vi "Phasor Explorer Update Parameters.vi"(8 "error in (no error)":errorcluster, 11 "VI in":refnum<vi>) -> (0 "error out":errorcluster, 1 "Detector Parameters":T12={"Frames/Image"=0, "Gates/Frame"=1, "Bits/Frame"=1, "Multiplicity"=0, "Incident Signal"=0.0, "Poisson Signal"=FALSE} {"Frames/Image" min=1; "Multiplicity" min=0; "Bits/Frame" min=1; "Gates/Frame" min=1}, 2 "Display Parameters":T10={"# Points"=1, "Ramp Type"=enum."Linear", "Type of Series"=enum."1-Exp Decays", "Min tau"=0.0, "Max tau"=0.0, "Include 0"=FALSE, "Include Infinity"=FALSE} {"Min tau" min=0.0; "Max tau" min=0.0; "# Points" min=1 step=1}, 3 "Decay & IRF Parameters":T8 {"Lifetime" min=0.0; "IRF Period" min=0.0}, 4 "tau*":dbl[unit], 5 "Gate Parameters":T5={"First Gate Start"=0.0, "Use Gate Center"=FALSE, "Gate Width"=0.0, "Gate Step"=0.0, "# Gates"=1.0, "Gate Type"=enum."Square", "Edge Width"=0.0, "Top Slope"=0.0, "Reversed Sawtooth?"=FALSE, "Analytical Computation"=FALSE, "Integration"=enum."Item 0", "Tolerance"=1.0, "# Steps"=1.0, "Type of User-defined Function"=enum."Gate", "Use Gate Step"=FALSE} {"# Steps" min=0.0; "Tolerance" min=0.0; "Top Slope" min=0.0; "Edge Width" min=0.0; "Gate Step" min=0.0; "# Gates" min=1.0 step=1.0; "Gate Width" min=0.0}, 6 "f0":dbl[unit], 7 "Phasor Parameters":T2={"Harmonic Frequency"=0.0, "Use f* = 1/D Frequency"=FALSE, "Calibrated Phasor"=FALSE, "Calibration Lifetime"=1e-09, "Phasor Calculation"=enum."Direct Sum", "SEPL Type"=enum."UC", "# Gates"=1.0, "Square Gate Width"=1e-09, "Show Ticks"=FALSE} {"Square Gate Width" min=0.0; "# Gates" min=0.0; "Calibration Lifetime" min=0.0; "Harmonic Frequency" min=0.0})   [LabVIEW 2019]
uses:
  Phasor Explorer Gate Parameter to Adjust.ctl
  Phasor Explorer Phasor Parameters.ctl
  Phasor Calculation Type.ctl
  SEPL Type.ctl
  Phasor Explorer Gate Parameters.ctl
  Gate Type.ctl
  Type of User-defined Function.ctl
  Phasor Explorer Decay Parameters.ctl
  IRF Model.ctl
  Phasor Explorer Display Parameters.ctl
  Type of Series.ctl
  Phasor Explorer Detector Parameters.ctl
panel:
  in  "Tab Control":T1(tab)
  in  "Edit User-defined Gate":bool
  in  "Gate Parameter to Adjust":T13 caption="Parameter to adjust"
  in  "Match Laser Period":bool
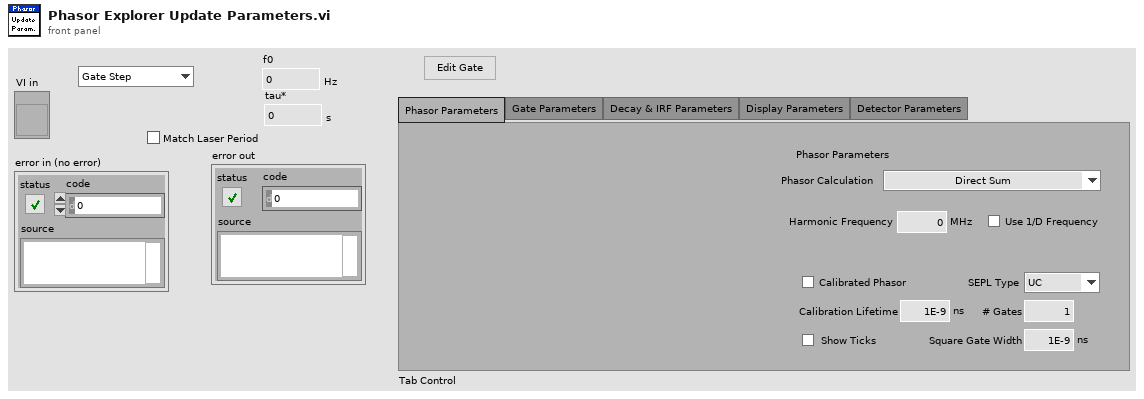
[diagram p1: front panel]
types:
  T1 = enum32{"Phasor Parameters", "Gate Parameters", "Decay & IRF Parameters", "Display Parameters", "Detector Parameters"}
  T2 = typedef "Phasor Explorer Phasor Parameters.ctl" = cluster{"Harmonic Frequency":dbl[unit], "Use f* = 1/D Frequency":bool, "Calibrated Phasor":bool, "Calibration Lifetime":dbl[unit], "Phasor Calculation":T3, "SEPL Type":T4, "# Gates":dbl, "Square Gate Width":dbl[unit], "Show Ticks":bool}
  T3 = typedef "Phasor Calculation Type.ctl" = enum16{"Direct Sum", "Analytical Formula"}
  T4 = typedef "SEPL Type.ctl" = enum16{"UC", "L_N", "L_N[W]", "L_X"}
  T5 = typedef "Phasor Explorer Gate Parameters.ctl" = cluster{"First Gate Start":dbl[unit], "Use Gate Center":bool, "Gate Width":dbl[unit], "Gate Step":dbl[unit], "# Gates":dbl, "Gate Type":T6, "Edge Width":dbl[unit], "Top Slope":dbl[unit], "Reversed Sawtooth?":bool, "Analytical Computation":bool, "Integration":enum32{"Item 0", "Item 1"}, "Tolerance":dbl, "# Steps":dbl, "Type of User-defined Function":T7, "Use Gate Step":bool}
  T6 = typedef "Gate Type.ctl" = enum16{"Square", "Finite Edge Square", "Finite Edge, Tilted Top Square", "Triangle", "Sawtooth", "User-defined"}
  T7 = typedef "Type of User-defined Function.ctl" = enum16{"Gate", "IRF"}
  T8 = typedef "Phasor Explorer Decay Parameters.ctl" = cluster{"Lifetime":dbl[unit], "IRF Offset":dbl[unit], "IRF Period":dbl[unit], "Normalized Decays":bool, "IRF Model":T9, "IRF Parameter 1":dbl[unit]}
  T9 = typedef "IRF Model.ctl" = enum16{"Dirac", "Exponential"}
  T10 = typedef "Phasor Explorer Display Parameters.ctl" = cluster{"# Points":i32, "Ramp Type":enum16{"Linear", "Logarithmic"}, "Type of Series":T11, "Min tau":dbl[unit], "Max tau":dbl[unit], "Include 0":bool, "Include Infinity":bool}
  T11 = typedef "Type of Series.ctl" = enum16{"1-Exp Decays", "Linear Combination of 1-Exp"}
  T12 = typedef "Phasor Explorer Detector Parameters.ctl" = cluster{"Frames/Image":i32, "Gates/Frame":i32, "Bits/Frame":i32, "Multiplicity":i32, "Incident Signal":dbl, "Poisson Signal":bool}
  T13 = typedef "Phasor Explorer Gate Parameter to Adjust.ctl" = enum16{"Gate Step", "# Gates"}
  T14 = typedef "SEPXP Gate Parameter to Adjust.ctl" = enum16{"Gate Step", "# Gates"}
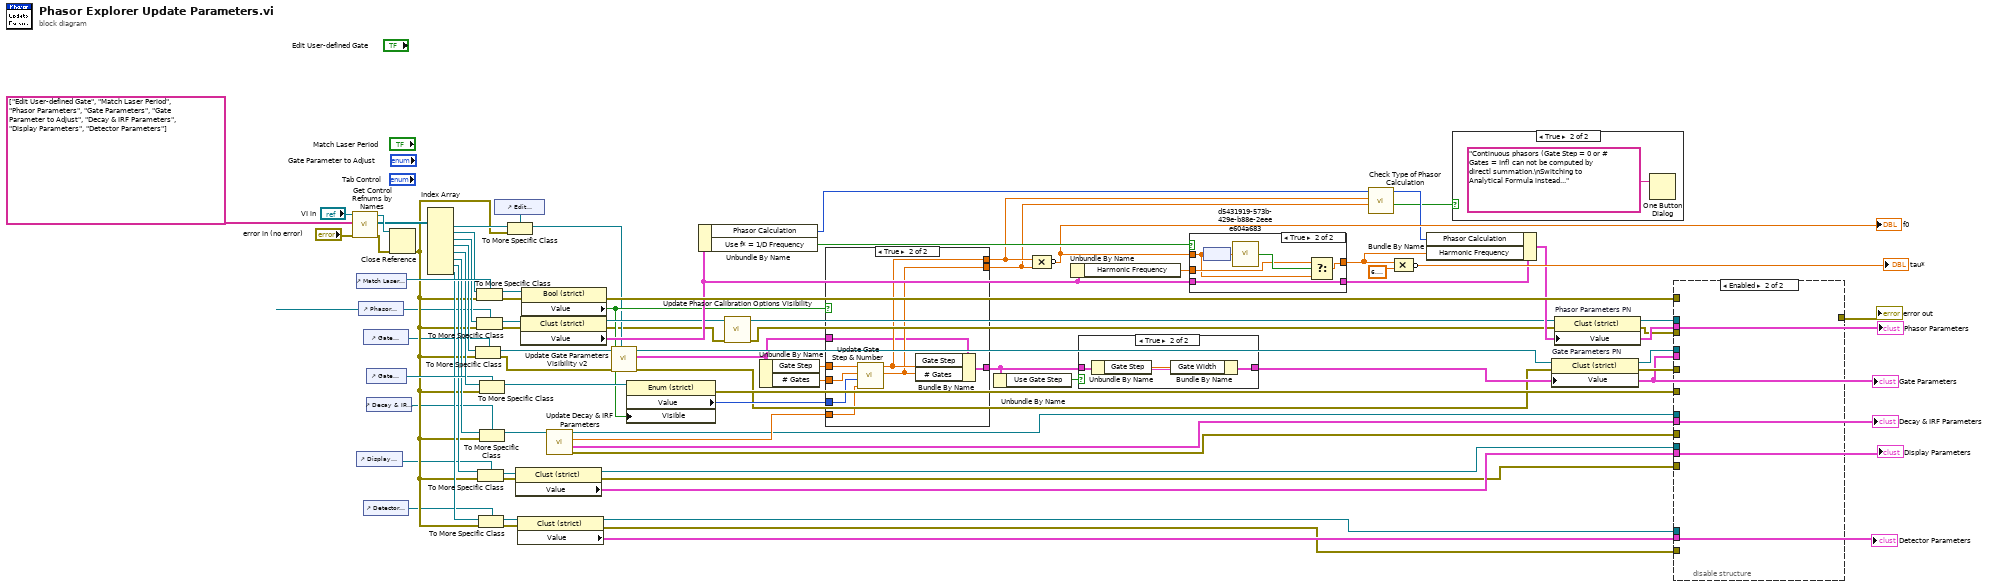
[diagram p0: block diagram]
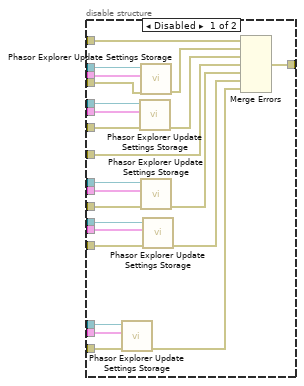
[diagram p2: hidden frame]
diagram:
  n1 = call "Get Control Refnums by Names.vi"("error in"="error in (no error)", "Control Labels"=string[] ["Edit User-defined Gate", "Match Laser Period", "Phasor Parameters", "Gate Parameters", "Gate Parameter to Adjust", "Decay & IRF Parameters", "Display Parameters", "Detector Parameters"], "VI  Ref"="VI in") -> ("error out"=w26:errorcluster, "Ctl Refnums"=w77:refnum<vi>[], "VI  Ref (out)"=w78:refnum<vi>)  [unwired: 5 in, 1 out]
  n2 = control-ref of="Match Laser Period"() -> (w72:refnum<vi>)
  n3 = control-ref of="Display Parameters"() -> (w6:refnum<vi>)
  n4 = control-ref of="Phasor Parameters"() -> (w9:refnum<vi>)
  n5 = control-ref of="Gate Parameters"() -> (w8:refnum<vi>)
  n6 = control-ref of="Detector Parameters"() -> (w5:refnum<vi>)
  n7 = control-ref of="Gate Parameter to Adjust"() -> (w66:refnum<vi>)
  n8 = control-ref of="Decay & IRF Parameters"() -> (w7:refnum<vi>)
  n9 = Close Reference(reference=w78, error in (no error)=w26) -> (error out=w21:errorcluster)
  n10 = Index Array(array=w77) -> (element #1=w25:refnum<vi>, element #2=w57:refnum<vi>, element #3=w56:refnum<vi>, element #4=w55:refnum<vi>, element #5=w68:refnum<vi>, element #6=w54:refnum<vi>, element #7=w41:refnum<vi>, element #8=w22:refnum<vi>)  [unwired: 8 in]
  n11 = To More Specific Class(target class=w8, reference=w55, error in=w21) -> (specific class reference=w61:refnum<vi>, error out=w60:errorcluster)
  n12 = To More Specific Class(target class=w72, reference=w57, error in=w21) -> (specific class reference=w71:refnum<vi>, error out=w70:errorcluster)
  n13 = To More Specific Class(target class=w9, reference=w56, error in=w21) -> (specific class reference=w63:refnum<vi>, error out=w62:errorcluster)
  n14 = To More Specific Class(target class=w6, reference=w41, error in=w21) -> (specific class reference=w40:refnum<vi>, error out=w39:errorcluster)
  n15 = To More Specific Class(target class=w5, reference=w22, error in=w21) -> (specific class reference=w20:refnum<vi>, error out=w19:errorcluster)
  n16 = To More Specific Class(target class=w66, reference=w68, error in=w21) -> (specific class reference=w67:refnum<vi>)  [unwired: 1 out]
  n17 = To More Specific Class(target class=w7, reference=w54, error in=w21) -> (specific class reference=w10:refnum<vi>)  [unwired: 1 out]
  n18 = control-ref of="Edit User-defined Gate"() -> (w24:refnum<vi>)
  n19 = To More Specific Class(target class=w24, reference=w25, error in=w21) -> (specific class reference=w23:refnum<vi>)  [unwired: 1 out]
  n20 = property class="Clust (strict)"(reference=w40, error in=w39) -> (reference out=w38:refnum<vi>, error out=w36:errorcluster, "Value"=w37:T10)
  "Display Parameters" <- w37
  n21 = property class="Clust (strict)"(reference=w20, error in=w19) -> (reference out=w18:refnum<vi>, error out=w16:errorcluster, "Value"=w17:T12)
  "Detector Parameters" <- w17
  n22 = property class="Clust (strict)"(reference=w63, error in=w62) -> (reference out=w30:refnum<vi>, error out=w4:errorcluster, "Value"=w46:T2)
  n23 = property class="Bool (strict)"(reference=w71, error in=w70) -> (error out=w69:errorcluster, "Value"=w27:bool)  [unwired: 1 out]
  n24 = call "Update Decay & IRF Parameters.vi"("Decay & IRF Parameters Refnum"=w10) -> ("error out"=w33:errorcluster, "Value"=w35:T8, "Laser Period"=w53:dbl[unit], "Decay & IRF Parameters Refnum"=w34:refnum<vi>)  [unwired: 7 in]
  "Decay & IRF Parameters" <- w35
  n25 = call "Update Gate Parameters Visibility v2.vi"("Edit User-defined Gate"=w23, "error in (no error)"=w60, "Gate Parameters in"=w61) -> ("error out"=w1:errorcluster, "Gate Parameters"=w2:T5, "Phasor Explorer Gate Parameters out"=w28:refnum<vi>)  [unwired: 6 in]
  n26 = property class="Enum (strict)"(reference=w67, "Visible"=w27) -> (error out=w64:errorcluster, "Value"=w65:T14)  [unwired: 1 in, 1 out]
  n27 = Unbundle By Name(w46) -> ("Phasor Calculation"=w32:T3, "Use f* = 1/D Frequency"=w76:bool)
  n28 = call "Update Phasor Calibration Options Visibility.vi"("Error In"=w4, "Phasor Explorer Phasor Parameters Refnum in"=w30) -> ("Error Out"=w3:errorcluster, "Phasor Explorer Phasor Parameters Refnum out"=w29:refnum<vi>)  [unwired: 8 in]
  n29 = Unbundle By Name(w2) -> ("Gate Step"=w59:dbl[unit], "# Gates"=w58:dbl)
  n30 = case shown="True" w27 {
    tunnel: w53 -> [_ w86]
    tunnel: [w84 w92] -> w51
    tunnel: [w83 w91] -> w50
    tunnel: w65 -> [_ w90]
    tunnel: w59 -> [w84 w89]
    tunnel: w58 -> [w83 w88]
    tunnel: w2 -> [w82 w87]
    tunnel: [w82 w85] -> w14
    frame False {
    }
    frame True {
      n31 = call "Update Gate Step & Number.vi"("Period"=w86, "Value to Update"=w90, "# Gates in"=w88, "Gate Step in"=w89) -> ("# Gates out"=w91:dbl, "Gate Step out"=w92:dbl[unit])  [unwired: 6 in]
      n32 = Bundle By Name(cluster=w87, "Gate Step"=w92, "# Gates"=w91) -> (w85:T5)
    }
  }
  n33 = Unbundle By Name(w14) -> ("Use Gate Step"=w15:bool)
  n34 = Compound Arithmetic op=MULTIPLY(w51, w50) -> (invert w47:dbl[unit])
  "f0" <- w47
  n35 = Unbundle By Name(w46) -> ("Harmonic Frequency"=w45:dbl[unit])
  n36 = case shown="True" w15 {
    tunnel: w14 -> [w93 w95]
    tunnel: [w93 w94] -> w13
    frame False {
    }
    frame True {
      n37 = Unbundle By Name(w95) -> ("Gate Step"=w96:dbl[unit])
      n38 = Bundle By Name(cluster=w95, "Gate Width"=w96) -> (w94:T5)
    }
  }
  "Gate Parameters" <- w13
  n39 = case shown="True" w76 {
    tunnel: w47 -> [_ w101]
    tunnel: [w97 w100] -> w12
    tunnel: w46 -> [w98 w104]
    tunnel: [w98 w104] -> w52
    tunnel: w45 -> [w97 w102]
    frame False {
    }
    frame True {
      # "update harmonic frequency"
      n40 = node(w101) -> (w99:dbl)
      n41 = call "d5431919-573b-429e-b88e-2eeee604a683.vi"("Number"=w99) -> ("Is NaN or Inf?"=w103:bool)  [unwired: 8 in]
      n42 = Select(t=w102, s=w103, f=w101) -> (s? t:f=w100:dbl[unit])
    }
  }
  n43 = call "Check Type of Phasor Calculation.vi"("# Gates"=w50, "Gate Step"=w51, "Phasor Calculation in"=w32) -> ("Changed?"=w11:bool, "Phasor Calculation out"=w31:T3)  [unwired: 7 in]
  n44 = Compound Arithmetic op=MULTIPLY(w12, 6.283185307179586) -> (invert →"tau*":dbl[unit])
  n45 = Bundle By Name(cluster=w52, "Phasor Calculation"=w31, "Harmonic Frequency"=w12) -> (w48:T2)
  "Phasor Parameters" <- w48
  n46 = case shown="True" w11 {
    frame False {
    }
    frame True {
      n47 = One Button Dialog(message="Continuous phasors (Gate Step = 0 or # Gates = Inf) can not be computed by directl summation.\nSwitching to Analytical Formula instead...") -> ()  [unwired: 1 in, 1 out]
    }
  }
  n48 = property on="Gate Parameters PN" class="Clust (strict)"(reference=w28, error in=w1, "Value"=w13) -> (reference out=w43:refnum<vi>, error out=w42:errorcluster)
  n49 = property on="Phasor Parameters PN" class="Clust (strict)"(reference=w29, error in=w3, "Value"=w48) -> (reference out=w49:refnum<vi>, error out=w44:errorcluster)
  n50 = disable-structure shown="Enabled" {
    disable-tunnel: [w128 _] -> w73
    disable-tunnel: w69 -> [w127 _]
    disable-tunnel: w64 -> [w126 _]
    disable-tunnel: w49 -> [w124 _]
    disable-tunnel: w48 -> [w123 _]
    disable-tunnel: w44 -> [w121 _]
    disable-tunnel: w43 -> [w120 _]
    disable-tunnel: w42 -> [w119 _]
    disable-tunnel: w38 -> [w116 _]
    disable-tunnel: w37 -> [w115 _]
    disable-tunnel: w36 -> [w114 _]
    disable-tunnel: w35 -> [w113 _]
    disable-tunnel: w34 -> [w112 _]
    disable-tunnel: w33 -> [w111 _]
    disable-tunnel: w18 -> [w110 _]
    disable-tunnel: w17 -> [w109 _]
    disable-tunnel: w16 -> [w108 _]
    disable-tunnel: w13 -> [w106 _]
    frame Disabled {
      n51 = call "Phasor Explorer Update Settings Storage.vi"("Error In"=w108, "NewVal"=w109, "CtlRef"=w110) -> ("Error Out"=w107:errorcluster)  [unwired: 8 in]
      n52 = call "Phasor Explorer Update Settings Storage.vi"("Error In"=w119, "NewVal"=w106, "CtlRef"=w120) -> ("Error Out"=w122:errorcluster)  [unwired: 8 in]
      n53 = call "Phasor Explorer Update Settings Storage.vi"("Error In"=w121, "NewVal"=w123, "CtlRef"=w124) -> ("Error Out"=w125:errorcluster)  [unwired: 8 in]
      n54 = call "Phasor Explorer Update Settings Storage.vi"("Error In"=w111, "NewVal"=w113, "CtlRef"=w112) -> ("Error Out"=w118:errorcluster)  [unwired: 8 in]
      n55 = call "Phasor Explorer Update Settings Storage.vi"("Error In"=w114, "NewVal"=w115, "CtlRef"=w116) -> ("Error Out"=w117:errorcluster)  [unwired: 8 in]
      n56 = Merge Errors(w127, w125, w122, w126, w118, w117, w107) -> (w128:errorcluster)
    }
    frame Enabled {
    }
  }
  "error out" <- w73
